vi "load_waveforms_for_script.vi"(8 "error in (no error)":errorcluster, 11 "HSDIO in":refnum<class "HSDIO.lvclass">) -> (0 "error out":errorcluster, 3 "HSDIO out":refnum<class "HSDIO.lvclass">)   [LabVIEW 2012, in "HSDIO.lvclass"]
uses:
  HSDIO.lvclass
  HSDIO.lvclass/HSDIO.ctl
  <vilib>/Utility/file.llb/Read From Spreadsheet File (string).vi
  <vilib>/regexp/Match Regular Expression.xnode
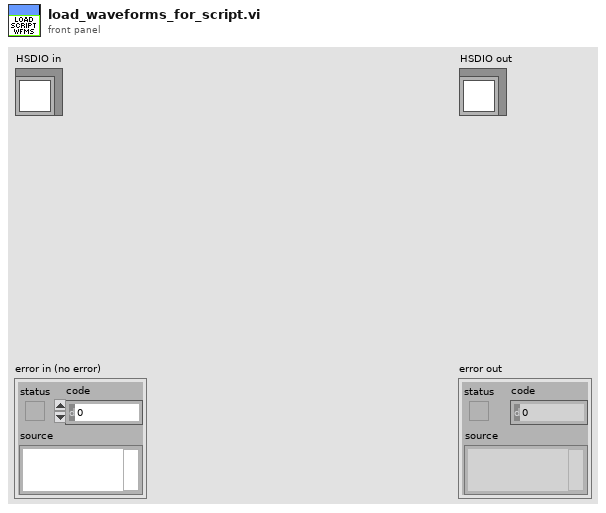
[diagram p1: front panel]
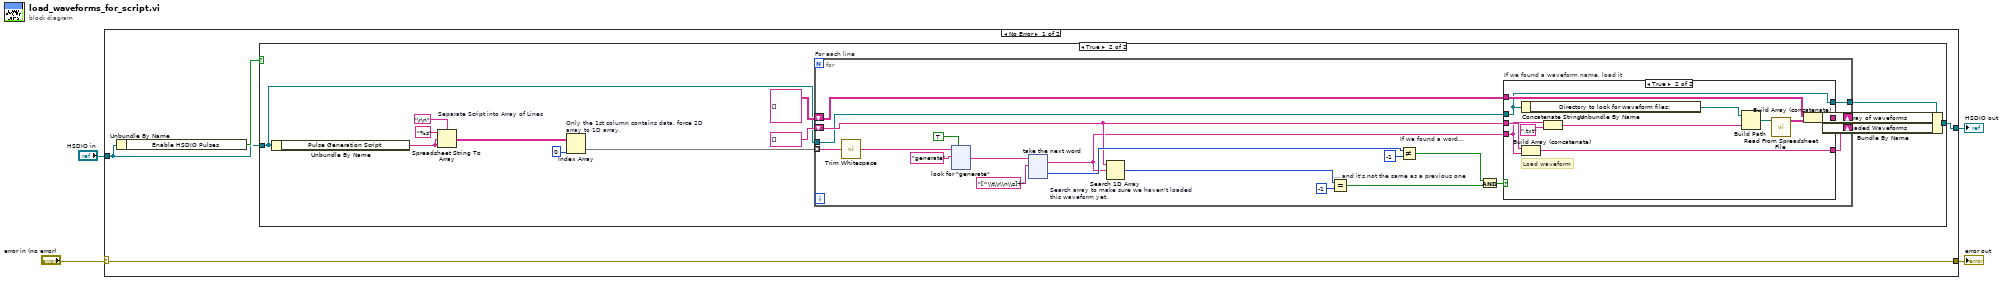
[diagram p0: block diagram]
diagram:
  n1 = case shown="No Error" "error in (no error)" {
    selector: "error in (no error)" -> [w8 w280]
    tunnel: [w8 w280] -> w3
    tunnel: [w5 w279] -> w1
    tunnel: "HSDIO in" -> [w6 w279]
    frame No Error {
      n2 = Unbundle By Name(w6) -> ("Enable HSDIO Pulses"=w7:bool)
      n3 = case shown="True" w7 {
        tunnel: w6 -> [w9 w14]
        tunnel: [w9 w12] -> w5
        frame False {
        }
        frame True {
          n4 = Unbundle By Name(w14) -> ("Pulse Generation Script"=w15:string)
          n5 = Spreadsheet String To Array "Separate Script into Array of Lines"(delimiter (Tab)="\r\n", format string="%s", spreadsheet string=w15, array type (2D Dbl)=w15) -> (array=w20:string[][])
          n6 = Index Array "Only the 1st column contains data, force 2D array to 1D array."(array=w20, index (col)=0 ("disabled index (col)")) -> (element=w18:string[])  [unwired: 1 in]
          n7 = for "For each line" {
            tunnel: w18 -> [w42] mode=indexing
            shift-right: [w34] -> w11
            shift-left: string[] [] -> [w31]
            shift-right: [w33] -> w10
            shift-left: string[][][] [] -> [w32]
            tunnel: w14 -> [w24]
            tunnel: [w23] -> w13
            n8 = call <vilib>:"Trim Whitespace.vi"("string"=w42) -> ("trimmed string"=w40:string)  [unwired: 1 in]
            n9 = xnode "look for \"generate\""("input string"=w40, "regular expression"="generate", "ignore case? (F)"=TRUE) -> ("after match"=w36:string)  [unwired: 3 in, 4 out]
            n10 = xnode "take the next word"("input string"=w36, "regular expression"="[^\\t\\r\\n\\s]+") -> ("whole match"=w30:string, "offset past match"=w35:i32)  [unwired: 4 in, 3 out]
            n11 = Search 1D Array "Search array to make sure we haven't loaded this waveform yet."(1D array=w31, element=w30) -> (index of element=w25:i32)  [unwired: 1 in]
            n12 = Equal? "... and it's not the same as a previous one"(x=w25, y=-1) -> (x = y?=w27:bool)
            n13 = Not Equal? "If we found a word..."(x=w35, y=-1) -> (x != y?=w28:bool)
            n14 = And(x=w28, y=w27) -> (x .and. y?=w26:bool)
            n15 = case "If we found a waveform name, load it" shown="True" w26 {
              tunnel: w30 -> [_ w51]
              tunnel: [w44 w48] -> w33
              tunnel: [w45 w53] -> w34
              tunnel: w31 -> [w45 w52]
              tunnel: w32 -> [w44 w50]
              tunnel: w24 -> [w43 w46]
              tunnel: [w43 w46] -> w23
              frame False {
                # "Don't load anything"
              }
              frame True {
                # "Load waveform"
                n16 = Unbundle By Name(w46) -> ("Directory to look for waveform files:"=w47:path)
                n17 = Build Array (concatenate)(w52, w51) -> (w53:string[])
                n18 = Concatenate Strings(w51, ".txt" ("string")) -> (w54:string)
                n19 = Build Path(base path=w47, name or relative path=w54) -> (appended path=w56:path)
                n20 = call-poly <vilib>:"Read From Spreadsheet File.vi"("file path (dialog if empty)"=w56) -> ("all rows"=w49:string[][])  [unwired: 6 in, 4 out]
                n21 = Build Array (concatenate)(w50, w49) -> (w48:string[][][])
              }
            }
          }
          n22 = Bundle By Name(cluster=w13, "array of waveforms"=w10, "Loaded Waveforms"=w11) -> (w12:refnum<class "HSDIO.lvclass">)
        }
      }
    }
    frame Error {
    }
  }
  "error out" <- w3
  "HSDIO out" <- w1
